vi "TecanCarvroPump_no delay.vi"(1 "Mode":T1(ring)=enum."Relative Dispense", 2 "TecanPump parameters":cluster{"Volume (μL)":u16, "Speed (μL/s)":u16}={"Volume (μL)"=100, "Speed (μL/s)"=30} {"Speed (μL/s)" min=1 max=5000 step=1; "Volume (μL)" max=5000 step=1}, 3 "Syringe size (μL)":u16=1000 min=1 max=5000 step=1, 4 "Valve":u8(knob)=6 max=6 step=1 scale=1.0..3.0, 5 "TecanPump address":u8 max=16 step=1, 6 "TecanPump COM":refnum<visa-resource-name>="COM6") -> (0 "Input string":string)   [LabVIEW 2023]
panel:
  out "Error out":errorcluster caption="错误输出"
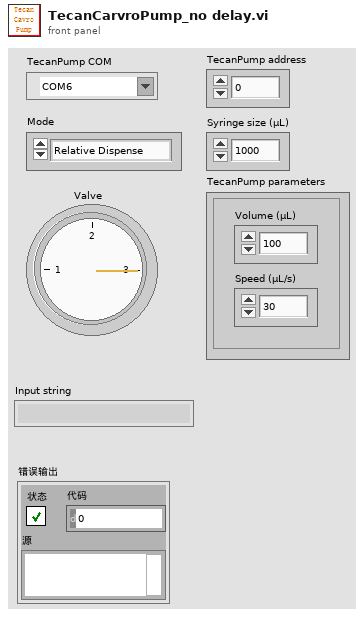
[diagram p1: front panel]
types:
  T1 = enum16{"Initialize", "Absolute Position", "Relative Pickup", "Relative Dispense", "Swich valve", "Bypass"}
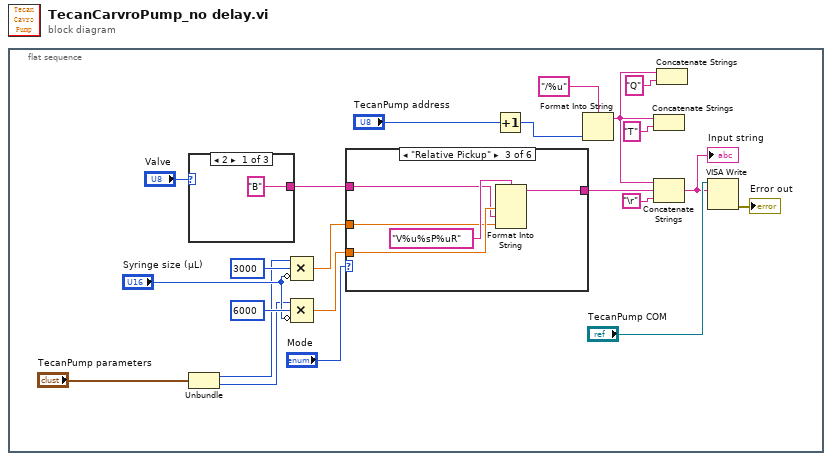
[diagram p0: block diagram]
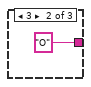
[diagram p2: hidden frame]
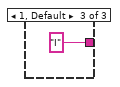
[diagram p3: hidden frame]
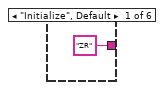
[diagram p4: hidden frame]
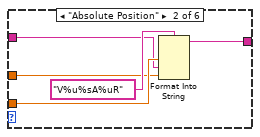
[diagram p5: hidden frame]
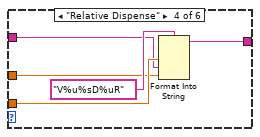
[diagram p6: hidden frame]
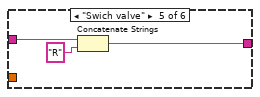
[diagram p7: hidden frame]
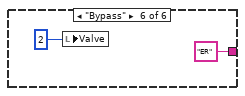
[diagram p8: hidden frame]
diagram:
  n1 = flat-sequence {
    frame #0 {
      n2 = case shown="2" "Valve" {
        tunnel: ["B" ("format string") "O" ("format string") "I" ("format string")] -> w10
        frame 2 {
        }
        frame 3 {
        }
        frame 1, Default {
        }
      }
      n3 = Unbundle("TecanPump parameters") -> ("Volume (μL)"=w3:u16, "Speed (μL/s)"=w2:u16)
      n4 = Compound Arithmetic op=MULTIPLY(w3, u16 3000 ("value"), invert "Syringe size (μL)") -> (w16:dbl)
      n5 = Compound Arithmetic op=MULTIPLY(w2, u16 6000 ("value"), invert "Syringe size (μL)") -> (w12:dbl)
      n6 = case shown="\"Relative Pickup\"" "Mode" {
        tunnel: w16 -> [_ w27 w33 w38 _ _]
        tunnel: w12 -> [_ w30 w35 w40 _ _]
        tunnel: ["ZR" w29 w34 w39 w42 "ER" ("string")] -> w11
        tunnel: w10 -> [_ w28 w32 w37 w44 _]
        frame "Initialize", Default {
        }
        frame "Absolute Position" {
          n7 = Format Into String(format string="V%u%sA%uR", w30, w28, w27) -> (resulting string=w29:string)  [unwired: 2 in, 1 out]
        }
        frame "Relative Pickup" {
          n8 = Format Into String(format string="V%u%sP%uR", w35, w32, w33) -> (resulting string=w34:string)  [unwired: 2 in, 1 out]
        }
        frame "Relative Dispense" {
          n9 = Format Into String(format string="V%u%sD%uR", w40, w37, w38) -> (resulting string=w39:string)  [unwired: 2 in, 1 out]
        }
        frame "Swich valve" {
          n10 = Concatenate Strings(w44, "R" ("string")) -> (w42:string)
        }
        frame "Bypass" {
          n11 = local write "Valve"(u8 2 ("Valve")) -> ()
        }
      }
      n12 = Increment(x="TecanPump address") -> (x+1=w17:u8)
      n13 = Format Into String(format string="/%u" ("字符串"), w17) -> (resulting string=w19:string)  [unwired: 2 in, 1 out]
      n14 = Concatenate Strings(w19, "T" ("字符串")) -> ()  [unwired: 1 out]
      n15 = Concatenate Strings(w19, w11, "\r") -> (w5:string)
      "Input string" <- w5
      n16 = Concatenate Strings(w19, "Q" ("字符串")) -> ()  [unwired: 1 out]
      n17 = VISA Write(VISA resource name="TecanPump COM", write buffer=w5) -> (error out=→"Error out":errorcluster)  [unwired: 1 in, 2 out]
    }
  }
